vi "Global demo.vi"() -> ()   [LabVIEW 2014]
panel:
  out "Demo PI Array":dbl[](array[numeric])=[20.0, 20.0, 20.0]
  out "Demo PI value":dbl
  out "demo":bool
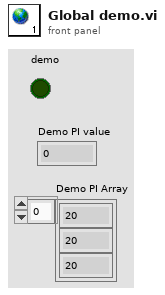
[diagram p1: front panel]
diagram:
